vi "varSCPI.vi"() -> ()   [LabVIEW 2020]
uses:
  controls/SCPI_enum.ctl
panel:
  in  "SCIPI":T1 items=["*IDN?"]
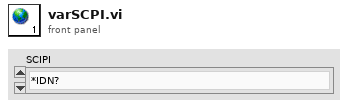
[diagram p1: front panel]
types:
  T1 = typedef "SCPI_enum.ctl" = u16
diagram:
